vi "Launch Logger.vi"(8 "error in (no error)":errorcluster, 11 "Historian Module in":refnum<class "Historian Module.lvclass">) -> (0 "error out":errorcluster, 3 "Historian Module out":refnum<class "Historian Module.lvclass">)   [LabVIEW 2020, in "VolatusHistorian.lvlib" / "Historian Module.lvclass"]
uses:
  Historian Module.lvclass
  Historian Module.lvclass/Historian Module.ctl
  Volatus/Module/Module.lvclass
  C:/dev/lv20CE/relink/lv-volatus/Volatus/Module/Module.lvclass
  C:/dev/lv20CE/relink/lv-volatus/VolatusHistorian/Historian Module/Historian Module.lvclass
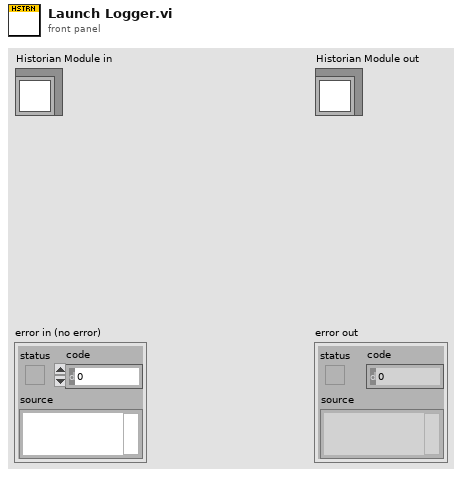
[diagram p1: front panel]
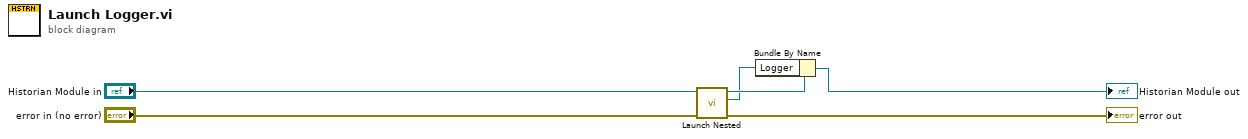
[diagram p0: block diagram]
diagram:
  n1 = call "Launch Nested.vi"("error in (no error)"="error in (no error)", "Parent in"="Historian Module in") -> ("error out"=→"error out":errorcluster, "MessageQ"=w1:refnum<class "MessageQ.lvclass">, "Parent out"=w3:refnum<class "Historian Module.lvclass">)  [unwired: 7 in]
  n2 = Bundle By Name(cluster=w3, "Logger"=w1) -> (→"Historian Module out":refnum<class "Historian Module.lvclass">)
